vi "test_F9P_232-2.vi"() -> ()   [LabVIEW 2019] (continued)
1*73\r\n$GBGSV,5,4,17,16,25,186,30,27,11,317,,28,62,307,37,33,76,249,24,1*7B\r\n$GBGSV,5,5,17,34,10,143,,1*40\r\n$GBGSV,5,1,17,01,42,153,,03,45,207,,04,35,133,,05,09,257,,3*7E\r\n$GBGSV,5,2,17,06,29,183,,07,07,201,,08,66,358,42,09,09,195,,3*7C\r\n$GBGSV,5,3,17,10,14,222,,11,34,144,,13,51,316,,14,73,036,46,3*70\r\n$GBGSV,5,4,17,16,25,186,33,27,11,317,,28,62,307,,33,76,249,,3*78\r\n$GBGSV,5,5,17,34,10,143,,3*42\r\n$GNGLL,3723.59652,N,12656.92463,E,065255.00,A,A*72\r\n$GNRMC,065256.00,A,3723.59660,N,12656.92463,E,0.025,,250720,,,A,V*16\r\n$GNVTG,,T,,M,0.025,N,0.047,K,A*39\r\n$GNGGA,065256.00,3723.59660,N,12656.92463,E,1,12,0.80,36.1,M,18.5,M,,*76\r\n$GNGSA,A,3,29,17,19,06,12,05,02,09,,,,,1.28,0.80,1.01,1*0C\r\n$GNGSA,A,3,85,71,72,,,,,,,,,,1.28,0.80,1.01,2*0F\r\n$GNGSA,A,3,36,19,11,04,09,12,,,,,,,1.28,0.80,1.01,3*03\r\n$GNGSA,A,3,28,11,14,10,33,08,,,,,,,1.28,0.80,1.01,4*01\r\n$GPGSV,4,1,13,02,69,341,33,04,05,036,09,05,51,267,38,06,55,084,32,1*67\r\n$GPGSV,4,2,13,07,08,101,,09,35,053,36,12,16,259,29,13,12,191,,1*6A\r\n$GPGSV,4,3,13,17,14,158,15,19,32,163,36,25,10,289,21,29,11,322,19,1*64\r\n$GPGSV,4,4,13,30,04,130,,1*53\r\n$GPGSV,4,1,13,02,69,341,,04,05,036,,05,51,267,34,06,55,084,34,6*63\r\n$GPGSV,4,2,13,07,08,101,19,09,35,053,36,12,16,259,,13,12,191,,6*6E\r\n$GPGSV,4,3,13,17,14,158,,19,32,163,,25,10,289,13,29,11,322,,6*6B\r\n$GPGSV,4,4,13,30,04,130,,6*54\r\n$GLGSV,2,1,06,70,49,030,,71,73,235,35,72,22,219,31,84,04,137,11,1*74\r\n$GLGSV,2,2,06,85,59,121,30,86,57,339,,1*7B\r\n$GLGSV,2,1,06,70,49,030,,71,73,235,40,72,22,219,16,84,04,137,12,3*72\r\n$GLGSV,2,2,06,85,59,121,33,86,57,339,,3*7A\r\n$GAGSV,3,1,09,02,02,284,09,04,67,075,28,05,01,213,,09,48,198,36,7*76\r\n$GAGSV,3,2,09,11,78,057,26,12,29,118,16,18,59,273,42,19,15,041,19,7*71\r\n$GAGSV,3,3,09,36,38,315,26,7*47\r\n$GAGSV,3,1,09,02,02,284,,04,67,075,40,05,01,213,,09,48,198,34,2*76\r\n$GAGSV,3,2,09,11,78,057,35,12,29,118,25,18,59,273,33,19,15,041,,2*78\r\n$GAGSV,3,3,09,36,38,315,17,2*40\r\n$GBGSV,5,1,17,01,42,153,,03,45,207,,04,35,133,,05,09,257,,1*7C\r\n$GBGSV,5,2,17,06,29,183,,07,07,201,,08,66,358,34,09,09,195,,1*7F\r\n$GBGSV,5,3,17,10,14,222,23,11,34,144,25,13,51,316,,14,73,036,35,1*70\r\n$GBGSV,5,4,17,16,25,186,30,27,11,317,,28,62,307,37,33,76,249,27,1*78\r\n$GBGSV,5,5,17,34,10,143,,1*40\r\n$GBGSV,5,1,17,01,42,153,,03,45,207,,04,35,133,,05,09,257,,3*7E\r\n$GBGSV,5,2,17,06,29,183,,07,07,201,,08,66,358,41,09,09,195,,3*7F\r\n$GBGSV,5,3,17,10,14,222,,11,34,144,,13,51,316,,14,73,036,44,3*72\r\n$GBGSV,5,4,17,16,25,186,32,27,11,317,,28,62,307,,33,76,249,,3*79\r\n$GBGSV,5,5,17,34,10,143,,3*42\r\n$GNGLL,3723.59660,N,12656.92463,E,065256.00,A,A*70\r\n$GNRMC,065257.00,A,3723.59674,N,12656.92461,E,0.007,,250720,,,A,V*10\r\n$GNVTG,,T,,M,0.007,N,0.013,K,A*38\r\n$GNGGA,065257.00,3723.59674,N,12656.92461,E,1,12,0.70,36.5,M,18.5,M,,*7B\r\n$GNGSA,A,3,29,17,19,06,12,05,02,09,,,,,1.18,0.70,0.95,1*0C\r\n$GNGSA,A,3,85,71,72,,,,,,,,,,1.18,0.70,0.95,2*0F\r\n$GNGSA,A,3,36,19,11,04,09,12,,,,,,,1.18,0.70,0.95,3*03\r\n$GNGSA,A,3,28,11,14,10,33,08,,,,,,,1.18,0.70,0.95,4*01\r\n$GPGSV,4,1,13,02,69,341,37,04,05,036,10,05,51,267,37,06,55,084,32,1*64\r\n$GPGSV,4,2,13,07,08,101,,09,35,053,36,12,16,259,29,13,12,191,,1*6A\r\n$GPGSV,4,3,13,17,14,158,15,19,32,163,36,25,10,289,21,29,11,322,19,1*64\r\n$GPGSV,4,4,13,30,04,130,,1*53\r\n$GPGSV,4,1,13,02,69,341,,04,05,036,,05,51,267,33,06,55,084,32,6*62\r\n$GPGSV,4,2,13,07,08,101,15,09,35,053,35,12,16,259,,13,12,191,,6*61\r\n$GPGSV,4,3,13,17,14,158,,19,32,163,,25,10,289,15,29,11,322,,6*6D\r\n$GPGSV,4,4,13,30,04,130,,6*54\r\n$GLGSV,2,1,06,70,49,030,,71,73,235,35,72,22,219,31,84,04,137,06,1*72\r\n$GLGSV,2,2,06,85,59,121,29,86,57,339,,1*73\r\n$GLGSV,2,1,06,70,49,030,,71,73,235,40,72,22,219,10,84,04,137,10,3*76\r\n$GLGSV,2,2,06,85,59,121,32,86,57,339,,3*7B\r\n$GAGSV,3,1,09,02,02,284,08,04,67,075,29,05,01,213,,09,48,198,36,7*76\r\n$GAGSV,3,2,09,11,78,057,26,12,29,118,16,18,59,273,42,19,14,041,19,7*70\r\n$GAGSV,3,3,09,36,38,315,26,7*47\r\n$GAGSV,3,1,09,02,02,284,,04,67,075,39,05,01,213,,09,48,198,34,2*78\r\n$GAGSV,3,2,09,11,78,057,34,12,29,118,26,18,59,273,34,19,14,041,,2*7C\r\n$GAGSV,3,3,09,36,38,315,18,2*4F\r\n$GBGSV,5,1,17,01,42,153,,03,45,207,,04,35,133,,05,09,257,,1*7C\r\n$GBGSV,5,2,17,06,29,183,,07,07,201,,08,66,358,34,09,09,195,,1*7F\r\n$GBGSV,5,3,17,10,14,222,23,11,34,144,25,13,51,316,,14,73,036,35,1*70\r\n$GBGSV,5,4,17,16,25,186,30,27,11,317,,28,62,307,37,33,76,249,29,1*76\r\n$GBGSV,5,5,17,34,10,143,,1*40\r\n$GBGSV,5,1,17,01,42,153,,03,45,207,,04,35,133,,05,09,257,,3*7E\r\n$GBGSV,5,2,17,06,29,183,,07,07,201,,08,66,358,40,09,09,195,,3*7E\r\n$GBGSV,5,3,17,10,14,222,,11,34,144,28,13,51,316,,14,73,036,42,3*7E\r\n$GBGSV,5,4,17,16,25,186,32,27,11,317,,28,62,307,,33,76,249,,3*79\r\n$GBGSV,5,5,17,34,10,143,,3*42\r\n$GNGLL,3723.59674,N,12656.92461,E,065257.00,A,A*76\r\n$GNRMC,065258.00,A,3723.59689,N,12656.92458,E,0.035,,250720,,,A,V*16\r\n$GNVTG,,T,,M,0.035,N,0.065,K,A*38\r\n$GNGGA,065258.00,3723.59689,N,12656.92458,E,1,12,0.70,37.0,M,18.5,M,,*78\r\n$GNGSA,A,3,29,17,19,06,12,05,02,09,,,,,1.18,0.70,0.95,1*0C\r\n$GNGSA,A,3,85,71,72,,,,,,,,,,1.18,0.70,0.95,2*0F\r\n$GNGSA,A,3,36,19,11,04,09,12,,,,,,,1.18,0.70,0.95,3*03\r\n$GNGSA,A,3,28,11,14,10,33,08,,,,,,,1.18,0.70,0.95,4*01\r\n$GPGSV,4,1,13,02,69,341,37,04,05,036,10,05,51,267,37,06,55,084,32,1*64\r\n$GPGSV,4,2,13,07,08,101,,09,35,053,35,12,16,259,29,13,12,191,,1*69\r\n$GPGSV,4,3,13,17,14,158,15,19,32,163,36,25,10,289,21,29,11,322,20,1*6E\r\n$GPGSV,4,4,13,30,04,130,,1*53\r\n$GPGSV,4,1,13,02,69,341,,04,05,036,,05,51,267,33,06,55,084,32,6*62\r\n$GPGSV,4,2,13,07,08,101,,09,35,053,35,12,16,259,,13,12,191,,6*65\r\n$GPGSV,4,3,13,17,14,158,,19,32,163,,25,10,289,15,29,11,322,,6*6D\r\n$GPGSV,4,4,13,30,04,130,,6*54\r\n$GLGSV,2,1,06,70,49,030,,71,73,235,35,72,22,219,31,84,04,137,06,1*72\r\n$GLGSV,2,2,06,85,59,121,26,86,57,339,,1*7C\r\n$GLGSV,2,1,06,70,49,030,,71,73,235,38,72,22,219,10,84,04,137,10,3*79\r\n$GLGSV,2,2,06,85,59,121,31,86,57,339,,3*78\r\n$GAGSV,3,1,09,02,02,284,09,04,67,075,29,05,01,213,,09,48,198,36,7*77\r\n$GAGSV,3,2,09,11,78,057,26,12,29,118,16,18,59,273,42,19,14,041,18,7*71\r\n$GAGSV,3,3,09,36,38,315,25,7*44\r\n$GAGSV,3,1,09,02,02,284,,04,67,075,39,05,01,213,,09,48,198,34,2*78\r\n$GAGSV,3,2,09,11,78,057,37,12,29,118,27,18,59,273,34,19,14,041,,2*7E\r\n$GAGSV,3,3,09,36,38,315,17,2*40\r\n$GBGSV,5,1,17,01,42,153,,03,45,207,,04,35,133,,05,09,257,,1*7C\r\n$GBGSV,5,2,17,06,29,183,,07,07,201,,08,66,358,34,09,09,195,,1*7F\r\n$GBGSV,5,3,17,10,14,222,23,11,34,144,25,13,51,316,,14,73,036,35,1*70\r\n$GBGSV,5,4,17,16,25,186,31,27,11,317,,28,62,307,37,33,76,249,29,1*77\r\n$GBGSV,5,5,17,34,10,143,,1*40\r\n$GBGSV,5,1,17,01,42,153,,03,45,207,,04,35,133,,05,09,257,,3*7E\r\n$GBGSV,5,2,17,06,29,183,,07,07,201,,08,66,358,40,09,09,195,,3*7E\r\n$GBGSV,5,3,17,10,14,222,,11,34,144,28,13,51,316,,14,73,036,42,3*7E\r\n$GBGSV,5,4,17,16,25,186,32,27,11,317,,28,62,307,,33,76,249,,3*79\r\n$GBGSV,5,5,17,34,10,143,,3*42\r\n$GNGLL,3723.59689,N,12656.92458,E,065258.00,A,A*71\r\n$GNRMC,065259.00,A,3723.59709,N,12656.92456,E,0.071,,250720,,,A,V*10\r\n$GNVTG,,T,,M,0.071,N,0.132,K,A*3B\r\n$GNGGA,065259.00,3723.59709,N,12656.92456,E,1,12,0.70,37.6,M,18.5,M,,*78\r\n$GNGSA,A,3,29,17,19,06,12,05,02,09,,,,,1.18,0.70,0.95,1*0C\r\n$GNGSA,A,3,85,71,72,,,,,,,,,,1.18,0.70,0.95,2*0F\r\n$GNGSA,A,3,36,19,11,04,09,12,,,,,,,1.18,0.70,0.95,3*03\r\n$GNGSA,A,3,28,11,14,10,33,08,,,,,,,1.18,0.70,0.95,4*01\r\n$GPGSV,4,1,13,02,69,341,36,04,05,036,12,05,51,267,37,06,55,084,32,1*67\r\n$GPGSV,4,2,13,07,08,101,,09,35,053,35,12,16,259,29,13,12,191,,1*69\r\n$GPGSV,4,3,13,17,14,158,15,19,32,163,36,25,10,289,20,29,11,322,19,1*65\r\n$GPGSV,4,4,13,30,04,130,,1*53\r\n$GPGSV,4,1,13,02,69,341,,04,05,036,,05,51,267,33,06,55,084,33,6*63\r\n$GPGSV,4,2,13,07,08,101,,09,35,053,35,12,16,259,,13,12,191,,6*65\r\n$GPGSV,4,3,13,17,14,158,,19,32,163,,25,10,289,15,29,11,322,,6*6D\r\n$GPGSV,4,4,13,30,04,130,,6*54\r\n$GLGSV,2,1,06,70,49,030,,71,73,235,35,72,22,219,31,84,04,137,12,1*77\r\n$GLGSV,2,2,06,85,59,121,23,86,57,339,,1*79\r\n$GLGSV,2,1,06,70,49,030,,71,73,235,38,72,22,219,14,84,04,137,10,3*7D\r\n$GLGSV,2,2,06,85,59,121,30,86,57,339,,3*79\r\n$GAGSV,3,1,09,02,02,284,09,04,67,075,29,05,01,213,,09,48,198,36,7*77\r\n$GAGSV,3,2,09,11,78,057,26,12,29,118,16,18,59,273,42,19,14,041,19,7*70\r\n$GAGSV,3,3,09,36,38,315,25,7*44\r\n$GAGSV,3,1,09,02,02,284,,04,67,075,39,05,01,213,,09,48,198,34,2*78\r\n$GAGSV,3,2,09,11,78,057,37,12,29,118,27,18,59,273,34,19,14,041,,2*7E\r\n$GAGSV,3,3,09,36,38,315,17,2*40\r\n$GBGSV,5,1,17,01,42,153,,03,45,207,,04,35,133,,05,09,257,,1*7C\r\n$GBGSV,5,2,17,06,29,183,,07,07,201,,08,66,358,34,09,09,195,,1*7F\r\n$GBGSV,5,3,17,10,14,222,24,11,34,144,25,13,51,316,,14,73,036,35,1*77\r\n$GBGSV,5,4,17,16,25,186,31,27,11,317,,28,62,307,37,33,76,249,28,1*76\r\n$GBGSV,5,5,17,34,10,143,,1*40\r\n$GBGSV,5,1,17,01,42,153,,03,45,207,,04,35,133,,05,09,257,,3*7E\r\n$GBGSV,5,2,17,06,29,183,,07,07,201,,08,66,358,40,09,09,195,,3*7E\r\n$GBGSV,5,3,17,10,14,222,,11,34,144,28,13,51,316,,14,73,036,43,3*7F\r\n$GBGSV,5,4,17,16,25,186,32,27,11,317,,28,62,307,,33,76,249,,3*79\r\n$GBGSV,5,5,17,34,10,143,,3*42\r\n$GNGLL,3723.59709,N,12656.92456,E,065259.00,A,A*77\r\n$GNRMC,065300.00,A,3723.59721,N,12656.92455,E,0.021,,250720,,,A,V*11\r\n$GNVTG,,T,,M,0.021,N,0.039,K,A*34\r\n$GNGGA,065300.00,3723.59721,N,12656.92455,E,1,12,0.78,38.0,M,18.5,M,,*7D\r\n$GNGSA,A,3,29,17,19,06,12,05,02,09,,,,,1.20,0.78,0.92,1*08\r\n$GNGSA,A,3,85,71,72,,,,,,,,,,1.20,0.78,0.92,2*0B\r\n$GNGSA,A,3,36,19,11,04,09,12,,,,,,,1.20,0.78,0.92,3*07\r\n$GNGSA,A,3,28,11,14,10,33,08,,,,,,,1.20,0.78,0.92,4*05\r\n$GPGSV,4,1,13,02,69,341,36,04,05,036,07,05,51,267,37,06,55,084,32,1*63\r\n$GPGSV,4,2,13,07,08,101,,09,35,053,35,12,16,259,28,13,12,191,,1*68\r\n$GPGSV,4,3,13,17,14,158,16,19,32,163,36,25,10,289,20,29,11,322,20,1*6C\r\n$GPGSV,4,4,13,30,04,130,,1*53\r\n$GPGSV,4,1,13,02,69,341,,04,05,036,,05,51,267,32,06,55,084,32,6*63\r\n$GPGSV,4,2,13,07,08,101,,09,35,053,32,12,16,259,,13,12,191,,6*62\r\n$GPGSV,4,3,13,17,14,158,,19,32,163,,25,10,289,15,29,11,322,,6*6D\r\n$GPGSV,4,4,13,30,04,130,,6*54\r\n$GLGSV,2,1,06,70,49,030,,71,73,235,35,72,22,219,31,84,04,137,09,1*7D\r\n$GLGSV,2,2,06,85,59,121,18,86,57,339,,1*71\r\n$GLGSV,2,1,06,70,49,030,,71,73,235,38,72,22,219,15,84,04,137,09,3*74\r\n$GLGSV,2,2,06,85,59,121,30,86,57,339,,3*79\r\n$GAGSV,3,1,09,02,02,284,09,04,67,075,30,05,01,213,,09,48,198,36,7*7F\r\n$GAGSV,3,2,09,11,78,057,26,12,29,118,18,18,59,273,43,19,14,041,18,7*7E\r\n$GAGSV,3,3,09,36,38,315,26,7*47\r\n$GAGSV,3,1,09,02,02,284,,04,67,075,39,05,01,213,,09,48,198,33,2*7F\r\n$GAGSV,3,2,09,11,78,057,35,12,29,118,28,18,59,273,35,19,14,041,,2*72\r\n$GAGSV,3,3,09,36,38,315,16,2*41\r\n$GBGSV,5,1,17,01,42,153,,03,45,207,,04,35,133,,05,09,257,,1*7C\r\n$GBGSV,5,2,17,06,29,183,,07,07,201,,08,66,358,34,09,09,195,,1*7F\r\n$GBGSV,5,3,17,10,14,222,23,11,34,144,25,13,51,316,,14,73,036,35,1*70\r\n$GBGSV,5,4,17,16,25,186,31,27,11,317,,28,62,307,37,33,76,249,28,1*76\r\n$GBGSV,5,5,17,34,10,143,,1*40\r\n$GBGSV,5,1,17,01,42,153,,03,45,207,,04,35,133,,05,09,257,,3*7E\r\n$GBGSV,5,2,17,06,29,183,,07,07,201,,08,66,358,39,09,09,195,,3*70\r\n$GBGSV,5,3,17,10,14,222,,11,34,144,28,13,51,316,,14,73,036,40,3*7C\r\n$GBGSV,5,4,17,16,25,186,31,27,11,317,,28,62,307,,33,76,249,,3*7A\r\n$GBGSV,5,5,17,34,10,143,,3*42\r\n$GNGLL,3723.59721,N,12656.92455,E,065300.00,A,A*73\r\n$GNRMC,065301.00,A,3723.59736,N,12656.92455,E,0.032,,250720,,,A,V*14\r\n$GNVTG,,T,,M,0.032,N,0.059,K,A*30\r\n$GNGGA,065301.00,3723.59736,N,12656.92455,E,1,12,0.72,38.4,M,18.5,M,,*74\r\n$GNGSA,A,3,29,17,19,06,12,05,02,09,,,,,1.15,0.72,0.90,1*06\r\n$GNGSA,A,3,85,71,72,,,,,,,,,,1.15,0.72,0.90,2*05\r\n$GNGSA,A,3,36,19,11,04,09,12,,,,,,,1.15,0.72,0.90,3*09\r\n$GNGSA,A,3,28,11,14,10,33,08,,,,,,,1.15,0.72,0.90,4*0B\r\n$GPGSV,4,1,13,02,69,341,33,04,05,036,08,05,51,267,37,06,55,084,33,1*68\r\n$GPGSV,4,2,13,07,08,101,,09,35,053,35,12,16,259,28,13,12,191,,1*68\r\n$GPGSV,4,3,13,17,14,158,15,19,32,163,36,25,10,289,21,29,11,322,21,1*6F\r\n$GPGSV,4,4,13,30,04,130,,1*53\r\n$GPGSV,4,1,13,02,69,341,,04,05,036,,05,51,267,33,06,55,084,35,6*65\r\n$GPGSV,4,2,13,07,08,101,,09,35,053,37,12,16,259,,13,12,191,,6*67\r\n$GPGSV,4,3,13,17,14,158,,19,32,163,,25,10,289,16,29,11,322,,6*6E\r\n$GPGSV,4,4,13,30,04,130,,6*54\r\n$GLGSV,2,1,06,70,49,030,,71,73,235,35,72,22,219,31,84,04,137,08,1*7C\r\n$GLGSV,2,2,06,85,59,121,17,86,57,339,,1*7E\r\n$GLGSV,2,1,06,70,49,030,,71,73,235,38,72,22,219,18,84,04,137,11,3*70\r\n$GLGSV,2,2,06,85,59,121,30,86,57,339,,3*79\r\n$GAGSV,3,1,09,02,02,284,11,04,67,075,30,05,01,213,,09,48,198,36,7*76\r\n$GAGSV,3,2,09,11,78,057,26,12,29,118,18,18,59,273,43,19,14,041,19,7*7F\r\n$GAGSV,3,3,09,36,38,315,26,7*47\r\n$GAGSV,3,1,09,02,02,284,,04,67,075,39,05,01,213,,09,48,198,33,2*7F\r\n$GAGSV,3,2,09,11,78,057,35,12,29,118,27,18,59,273,34,19,14,041,,2*7C\r\n$GAGSV,3,3,09,36,38,315,15,2*42\r\n$GBGSV,5,1,17,01,42,153,,03,45,207,,04,35,133,,05,09,257,,1*7C\r\n$GBGSV,5,2,17,06,29,183,,07,07,201,,08,66,358,33,09,09,195,,1*78\r\n$GBGSV,5,3,17,10,14,222,24,11,34,144,25,13,51,316,,14,73,036,35,1*77\r\n$GBGSV,5,4,17,16,25,186,31,27,11,317,,28,62,307,36,33,76,249,29,1*76\r\n$GBGSV,5,5,17,34,10,143,,1*40\r\n$GBGSV,5,1,17,01,42,153,,03,45,207,,04,35,133,,05,09,257,,3*7E\r\n$GBGSV,5,2,17,06,29,183,,07,07,201,,08,66,358,39,09,09,195,,3*70\r\n$GBGSV,5,3,17,10,14,222,,11,34,144,27,13,51,316,,14,73,036,43,3*70\r\n$GBGSV,5,4,17,16,25,186,31,27,11,317,,28,62,307,,33,76,249,,3*7A\r\n$GBGSV,5,5,17,34,10,143,,3*42\r\n$GNGLL,3723.59736,N,12656.92455,E,065301.00,A,A*74\r\n$GNRMC,065302.00,A,3723.59754,N,12656.92453,E,0.052,,250720,,,A,V*13\r\n$GNVTG,,T,,M,0.052,N,0.096,K,A*35\r\n$GNGGA,065302.00,3723.59754,N,12656.92453,E,1,12,0.72,38.8,M,18.5,M,,*79\r\n$GNGSA,A,3,29,17,19,06,12,05,02,09,,,,,1.15,0.72,0.90,1*06\r\n$GNGSA,A,3,85,71,72,,,,,,,,,,1.15,0.72,0.90,2*05\r\n$GNGSA,A,3,36,19,11,04,09,12,,,,,,,1.15,0.72,0.90,3*09\r\n$GNGSA,A,3,28,11,14,10,33,08,,,,,,,1.15,0.72,0.90,4*0B\r\n$GPGSV,4,1,13,02,69,341,34,04,05,036,08,05,51,267,37,06,55,084,33,1*6F\r\n$GPGSV,4,2,13,07,08,101,,09,35,053,35,12,16,259,28,13,12,191,,1*68\r\n$GPGSV,4,3,13,17,14,158,14,19,32,163,36,25,10,289,22,29,11,322,21,1*6D\r\n$GPGSV,4,4,13,30,04,130,,1*53\r\n$GPGSV,4,1,13,02,69,341,,04,05,036,,05,51,267,32,06,55,084,31,6*60\r\n$GPGSV,4,2,13,07,08,101,,09,35,053,34,12,16,259,,13,12,191,,6*64\r\n$GPGSV,4,3,13,17,14,158,,19,32,163,,25,10,289,16,29,11,322,,6*6E\r\n$GPGSV,4,4,13,30,04,130,,6*54\r\n$GLGSV,2,1,06,70,49,030,,71,73,235,35,72,22,219,31,84,04,137,08,1*7C\r\n$GLGSV,2,2,06,85,59,121,21,86,57,339,,1*7B\r\n$GLGSV,2,1,06,70,49,030,,71,73,235,36,72,22,219,19,84,04,137,10,3*7E\r\n$GLGSV,2,2,06,85,59,121,29,86,57,339,,3*71\r\n$GAGSV,3,1,09,02,02,284,08,04,67,075,29,05,01,213,,09,48,198,36,7*76\r\n$GAGSV,3,2,09,11,78,057,26,12,29,118,19,18,59,273,43,19,14,041,19,7*7E\r\n$GAGSV,3,3,09,36,38,315,26,7*47\r\n$GAGSV,3,1,09,02,02,284,,04,67,075,38,05,01,213,,09,48,198,34,2*79\r\n$GAGSV,3,2,09,11,78,057,36,12,29,118,28,18,59,273,31,19,14,041,,2*75\r\n$GAGSV,3,3,09,36,38,315,16,2*41\r\n$GBGSV,5,1,17,01,42,153,,03,45,207,,04,35,133,,05,09,257,,1*7C\r\n$GBGSV,5,2,17,06,29,183,,07,07,201,,08,66,358,33,09,09,195,,1*78\r\n$GBGSV,5,3,17,10,14,222,24,11,34,144,24,13,51,316,,14,73,036,35,1*76\r\n$GBGSV,5,4,17,16,25,186,31,27,11,317,,28,62,307,37,33,76,249,28,1*76\r\n$GBGSV,5,5,17,34,10,143,,1*40\r\n$GBGSV,5,1,17,01,42,153,,03,45,207,,04,35,133,,05,09,257,,3*7E\r\n$GBGSV,5,2,17,06,29,183,,07,07,201,,08,66,358,38,09,09,195,,3*71\r\n$GBGSV,5,3,17,10,14,222,,11,34,144,27,13,51,316,,14,73,036,41,3*72\r\n$GBGSV,5,4,17,16,25,186,31,27,11,317,,28,62,307,,33,76,249,,3*7A\r\n$GBGSV,5,5,17,34,10,143,,3*42\r\n$GNGLL,3723.59754,N,12656.92453,E,065302.00,A,A*75\r\n$GNRMC,065303.00,A,3723.59771,N,12656.92452,E,0.013,,250720,,,A,V*11\r\n$GNVTG,,T,,M,0.013,N,0.023,K,A*3E\r\n$GNGGA,065303.00,3723.59771,N,12656.92452,E,1,12,0.72,39.1,M,18.5,M,,*76\r\n$GNGSA,A,3,29,17,19,06,12,05,02,09,,,,,1.15,0.72,0.90,1*06\r\n$GNGSA,A,3,85,71,72,,,,,,,,,,1.15,0.72,0.90,2*05\r\n$GNGSA,A,3,36,19,11,04,09,12,,,,,,,1.15,0.72,0.90,3*09\r\n$GNGSA,A,3,28,11,14,10,33,08,,,,,,,1.15,0.72,0.90,4*0B\r\n$GPGSV,4,1,13,02,69,341,33,04,05,036,09,05,51,267,38,06,55,084,33,1*66\r\n$GPGSV,4,2,13,07,08,101,,09,35,053,35,12,16,259,27,13,12,191,,1*67\r\n$GPGSV,4,3,13,17,14,158,14,19,32,163,36,25,10,289,22,29,11,322,22,1*6E\r\n$GPGSV,4,4,13,30,04,130,,1*53\r\n$GPGSV,4,1,13,02,69,341,,04,05,036,,05,51,267,32,06,55,084,37,6*66\r\n$GPGSV,4,2,13,07,08,101,,09,35,053,37,12,16,259,,13,12,191,,6*67\r\n$GPGSV,4,3,13,17,14,158,,19,32,163,,25,10,289,16,29,11,322,,6*6E\r\n$GPGSV,4,4,13,30,04,130,,6*54\r\n$GLGSV,2,1,06,70,49,030,,71,73,235,36,72,22,219,31,84,04,137,11,1*77\r\n$GLGSV,2,2,06,85,59,121,25,86,57,339,,1*7F\r\n$GLGSV,2,1,06,70,49,030,,71,73,235,37,72,22,219,13,84,04,137,09,3*7D\r\n$GLGSV,2,2,06,85,59,121,28,86,57,339,,3*70\r\n$GAGSV,3,1,09,02,02,284,07,04,67,075,29,05,01,213,,09,48,198,36,7*79\r\n$GAGSV,3,2,09,11,78,057,26,12,29,118,21,18,59,273,43,19,14,041,18,7*74\r\n$GAGSV,3,3,09,36,38,315,26,7*47\r\n$GAGSV,3,1,09,02,02,284,,04,67,075,40,05,01,213,,09,48,198,33,2*71\r\n$GAGSV,3,2,09,11,78,057,36,12,29,118,28,18,59,273,32,19,14,041,,2*76\r\n$GAGSV,3,3,09,36,38,315,17,2*40\r\n$GBGSV,5,1,17,01,42,153,,03,45,207,,04,35,133,,05,09,257,,1*7C\r\n$GBGSV,5,2,17,06,29,183,,07,07,201,,08,66,358,33,09,09,195,,1*78\r\n$GBGSV,5,3,17,10,14,222,23,11,34,144,23,13,51,316,,14,73,036,35,1*76\r\n$GBGSV,5,4,17,16,25,186,31,27,11,317,,28,62,307,37,33,76,249,29,1*77\r\n$GBGSV,5,5,17,34,10,143,,1*40\r\n$GBGSV,5,1,17,01,42,153,,03,45,207,,04,35,133,,05,09,257,,3*7E\r\n$GBGSV,5,2,17,06,29,183,,07,07,201,,08,66,358,39,09,09,195,,3*70\r\n$GBGSV,5,3,17,10,14,222,,11,34,144,27,13,51,316,,14,73,036,43,3*70\r\n$GBGSV,5,4,17,16,25,186,32,27,11,317,,28,62,307,,33,76,249,,3*79\r\n$GBGSV,5,5,17,34,10,143,,3*42\r\n$GNGLL,3723.59771,N,12656.92452,E,065303.00,A,A*72\r\n$GNRMC,065304.00,A,3723.59784,N,12656.92450,E,0.021,,250720,,,A,V*1F\r\n$GNVTG,,T,,M,0.021,N,0.039,K,A*34\r\n$GNGGA,065304.00,3723.59784,N,12656.92450,E,1,12,0.78,39.4,M,18.5,M,,*76\r\n$GNGSA,A,3,29,17,19,06,12,05,02,09,,,,,1.20,0.78,0.92,1*08\r\n$GNGSA,A,3,85,71,72,,,,,,,,,,1.20,0.78,0.92,2*0B\r\n$GNGSA,A,3,36,19,11,04,09,12,,,,,,,1.20,0.78,0.92,3*07\r\n$GNGSA,A,3,28,11,14,10,33,08,,,,,,,1.20,0.78,0.92,4*05\r\n$GPGSV,4,1,13,02,69,341,33,04,05,036,09,05,51,267,38,06,55,084,33,1*66\r\n$GPGSV,4,2,13,07,08,101,,09,35,053,35,12,16,259,27,13,12,191,,1*67\r\n$GPGSV,4,3,13,17,14,158,13,19,32,163,36,25,10,289,22,29,11,322,22,1*69\r\n$GPGSV,4,4,13,30,04,130,,1*53\r\n$GPGSV,4,1,13,02,69,341,,04,05,036,,05,51,267,33,06,55,084,34,6*64\r\n$GPGSV,4,2,13,07,08,101,,09,35,053,37,12,16,259,,13,12,191,,6*67\r\n$GPGSV,4,3,13,17,14,158,,19,32,163,,25,10,289,17,29,11,322,,6*6F\r\n$GPGSV,4,4,13,30,04,130,,6*54\r\n$GLGSV,2,1,06,70,49,030,,71,73,235,35,72,22,219,30,84,04,137,09,1*7C\r\n$GLGSV,2,2,06,85,59,121,27,86,57,339,,1*7D\r\n$GLGSV,2,1,06,70,49,030,,71,73,235,37,72,22,219,16,84,04,137,08,3*79\r\n$GLGSV,2,2,06,85,59,121,28,86,57,339,,3*70\r\n$GAGSV,3,1,09,02,02,284,08,04,67,075,29,05,01,213,,09,48,198,36,7*76\r\n$GAGSV,3,2,09,11,78,057,26,12,29,118,22,18,59,273,43,19,14,041,18,7*77\r\n$GAGSV,3,3,09,36,38,315,26,7*47\r\n$GAGSV,3,1,09,02,02,284,,04,67,075,40,05,01,213,,09,48,198,33,2*71\r\n$GAGSV,3,2,09,11,78,057,36,12,29,118,27,18,59,273,32,19,14,041,,2*79\r\n$GAGSV,3,3,09,36,38,315,18,2*4F\r\n$GBGSV,5,1,17,01,42,153,,03,45,207,,04,35,133,,05,09,257,,1*7C\r\n$GBGSV,5,2,17,06,29,183,,07,07,201,,08,66,358,33,09,09,195,,1*78\r\n$GBGSV,5,3,17,10,14,222,23,11,34,144,23,13,51,316,,14,73,036,35,1*76\r\n$GBGSV,5,4,17,16,25,186,31,27,11,317,,28,62,307,37,33,76,249,29,1*77\r\n$GBGSV,5,5,17,34,10,143,,1*40\r\n$GBGSV,5,1,17,01,42,153,,03,45,207,,04,35,133,,05,09,257,,3*7E\r\n$GBGSV,5,2,17,06,29,183,,07,07,201,,08,66,358,40,09,09,195,,3*7E\r\n$GBGSV,5,3,17,10,14,222,,11,34,144,27,13,51,316,,14,73,036,43,3*70\r\n$GBGSV,5,4,17,16,25,186,32,27,11,317,,28,62,307,,33,76,249,,3*79\r\n$GBGSV,5,5,17,34,10,143,,3*42\r\n$GNGLL,3723.59784,N,12656.92450,E,065304.00,A,A*7D\r\n$GNRMC,065305.00,A,3723.59802,N,12656.92448,E,0.045,,250720,,,A,V*14\r\n$GNVTG,,T,,M,0.045,N,0.084,K,A*30\r\n$GNGGA,065305.00,3723.59802,N,12656.92448,E,1,12,0.72,39.8,M,18.5,M,,*79\r\n$GNGSA,A,3,29,17,19,06,12,05,02,09,,,,,1.15,0.72,0.90,1*06\r\n$GNGSA,A,3,85,71,72,,,,,,,,,,1.15,0.72,0.90,2*05\r\n$GNGSA,A,3,36,19,11,04,09,12,,,,,,,1.15,0.72,0.90,3*09\r\n$GNGSA,A,3,28,11,14,10,33,08,,,,,,,1.15,0.72,0.90,4*0B\r\n$GPGSV,4,1,13,02,69,341,36,04,05,036,11,05,51,267,38,06,55,084,34,1*6D\r\n$GPGSV,4,2,13,07,08,101,,09,35,053,35,12,16,259,26,13,12,191,17,1*60\r\n$GPGSV,4,3,13,17,14,158,14,19,32,163,36,25,10,289,22,29,11,322,22,1*6E\r\n$GPGSV,4,4,13,30,04,130,,1*53\r\n$GPGSV,4,1,13,02,69,341,,04,05,036,,05,51,267,33,06,55,084,32,6*62\r\n$GPGSV,4,2,13,07,08,101,,09,35,053,34,12,16,259,,13,12,191,,6*64\r\n$GPGSV,4,3,13,17,14,158,,19,32,163,,25,10,289,17,29,11,322,,6*6F\r\n$GPGSV,4,4,13,30,04,130,,6*54\r\n$GLGSV,2,1,06,70,49,030,,71,73,235,36,72,22,219,30,84,04,137,10,1*77\r\n$GLGSV,2,2,06,85,59,121,30,86,57,339,,1*7B\r\n$GLGSV,2,1,06,70,49,030,,71,73,235,37,72,22,219,18,84,04,137,08,3*77\r\n$GLGSV,2,2,06,85,59,121,29,86,57,339,,3*71\r\n$GAGSV,3,1,09,02,02,284,09,04,67,075,29,05,01,213,,09,48,198,36,7*77\r\n$GAGSV,3,2,09,11,78,057,27,12,29,118,23,18,59,273,43,19,14,041,17,7*78\r\n$GAGSV,3,3,09,36,38,315,27,7*46\r\n$GAGSV,3,1,09,02,02,284,,04,67,075,39,05,01,213,,09,48,198,33,2*7F\r\n$GAGSV,3,2,09,11,78,057,36,12,29,118,27,18,59,273,33,19,14,041,,2*78\r\n$GAGSV,3,3,09,36,38,315,18,2*4F\r\n$GBGSV,5,1,17,01,42,153,,03,45,207,,04,35,133,,05,09,257,,1*7C\r\n$GBGSV,5,2,17,06,29,183,,07,07,201,,08,66,358,33,09,09,195,,1*78\r\n$GBGSV,5,3,17,10,14,222,23,11,34,144,22,13,51,316,,14,73,036,35,1*77\r\n$GBGSV,5,4,17,16,25,186,31,27,11,317,,28,62,307,37,33,76,249,29,1*77\r\n$GBGSV,5,5,17,34,10,143,,1*40\r\n$GBGSV,5,1,17,01,42,153,,03,45,207,,04,35,133,,05,09,257,,3*7E\r\n$GBGSV,5,2,17,06,29,183,,07,07,201,,08,66,358,40,09,09,195,,3*7E\r\n$GBGSV,5,3,17,10,14,222,,11,34,144,28,13,51,316,,14,73,036,43,3*7F\r\n$GBGSV,5,4,17,16,25,186,32,27,11,317,,28,62,307,,33,76,249,,3*79\r\n$GBGSV,5,5,17,34,10,143,,3*42\r\n$GNGLL,3723.59802,N,12656.92448,E,065305.00,A,A*74\r\n$GNRMC,065306.00,A,3723.59821,N,12656.92443,E,0.051,,250720,,,A,V*18\r\n$GNVTG,,T,,M,0.051,N,0.094,K,A*34\r\n$GNGGA,065306.00,3723.59821,N,12656.92443,E,1,12,0.72,40.2,M,18.5,M,,*74\r\n$GNGSA,A,3,29,17,19,06,12,05,02,09,,,,,1.15,0.72,0.90,1*06\r\n$GNGSA,A,3,85,71,72,,,,,,,,,,1.15,0.72,0.90,2*05\r\n$GNGSA,A,3,36,19,11,04,09,12,,,,,,,1.15,0.72,0.90,3*09\r\n$GNGSA,A,3,28,11,14,10,33,08,,,,,,,1.15,0.72,0.90,4*0B\r\n$GPGSV,4,1,13,02,69,341,36,04,05,036,12,05,51,267,38,06,55,084,34,1*6E\r\n$GPGSV,4,2,13,07,08,101,,09,35,053,35,12,16,259,26,13,12,191,17,1*60\r\n$GPGSV,4,3,13,17,14,158,16,19,32,163,36,25,10,289,22,29,11,322,22,1*6C\r\n$GPGSV,4,4,13,30,04,130,,1*53\r\n$GPGSV,4,1,13,02,69,341,,04,05,036,,05,51,267,33,06,55,084,32,6*62\r\n$GPGSV,4,2,13,07,08,101,,09,35,053,35,12,16,259,,13,12,191,,6*65\r\n$GPGSV,4,3,13,17,14,158,,19,32,163,,25,10,289,17,29,11,322,,6*6F\r\n$GPGSV,4,4,13,30,04,130,,6*54\r\n$GLGSV,2,1,06,70,49,030,,71,73,235,36,72,22,219,30,84,04,137,11,1*76\r\n$GLGSV,2,2,06,85,59,121,31,86,57,339,,1*7A\r\n$GLGSV,2,1,06,70,49,030,,71,73,235,37,72,22,219,19,84,04,137,09,3*77\r\n$GLGSV,2,2,06,85,59,121,29,86,57,339,,3*71\r\n$GAGSV,3,1,09,02,02,284,07,04,67,075,29,05,01,213,,09,48,198,35,7*7A\r\n$GAGSV,3,2,09,11,78,057,27,12,29,118,25,18,59,273,43,19,14,041,18,7*71\r\n$GAGSV,3,3,09,36,38,315,26,7*47\r\n$GAGSV,3,1,09,02,02,284,,04,67,075,40,05,01,213,,09,48,198,33,2*71\r\n$GAGSV,3,2,09,11,78,057,36,12,29,118,27,18,59,273,33,19,14,041,,2*78\r\n$GAGSV,3,3,09,36,38,315,19,2*4E\r\n$GBGSV,5,1,17,01,42,153,,03,45,207,,04,35,133,,05,09,257,,1*7C\r\n$GBGSV,5,2,17,06,29,183,,07,07,201,,08,66,358,33,09,09,195,,1*78\r\n$GBGSV,5,3,17,10,14,222,23,11,34,144,22,13,51,316,,14,73,036,35,1*77\r\n$GBGSV,5,4,17,16,25,186,31,27,11,317,,28,62,307,38,33,76,249,28,1*79\r\n$GBGSV,5,5,17,34,10,143,,1*40\r\n$GBGSV,5,1,17,01,42,153,,03,45,207,,04,35,133,,05,09,257,,3*7E\r\n$GBGSV,5,2,17,06,29,183,,07,07,201,,08,66,358,40,09,09,195,,3*7E\r\n$GBGSV,5,3,17,10,14,222,,11,34,144,28,13,51,316,,14,73,036,43,3*7F\r\n$GBGSV,5,4,17,16,25,186,32,27,11,317,,28,62,307,,33,76,249,,3*79\r\n$GBGSV,5,5,17,34,10,143,,3*42\r\n$GNGLL,3723.59821,N,12656.92443,E,065306.00,A,A*7D\r\n$GNRMC,065307.00,A,3723.59840,N,12656.92439,E,0.036,,250720,,,A,V*12\r\n$GNVTG,,T,,M,0.036,N,0.066,K,A*38\r\n$GNGGA,065307.00,3723.59840,N,12656.92439,E,1,12,0.72,40.5,M,18.5,M,,*78\r\n$GNGSA,A,3,29,17,19,06,12,05,02,09,,,,,1.15,0.72,0.90,1*06\r\n$GNGSA,A,3,85,71,72,,,,,,,,,,1.15,0.72,0.90,2*05\r\n$GNGSA,A,3,36,19,11,04,09,12,,,,,,,1.15,0.72,0.90,3*09\r\n$GNGSA,A,3,28,11,14,10,33,08,,,,,,,1.15,0.72,0.90,4*0B\r\n$GPGSV,4,1,13,02,69,341,37,04,05,036,13,05,51,267,38,06,55,084,35,1*6F\r\n$GPGSV,4,2,13,07,08,101,,09,35,053,35,12,16,259,26,13,12,191,18,1*6F\r\n$GPGSV,4,3,13,17,14,158,16,19,32,163,36,25,10,289,22,29,11,322,23,1*6D\r\n$GPGSV,4,4,13,30,04,130,,1*53\r\n$GPGSV,4,1,13,02,69,341,,04,05,036,,05,51,267,33,06,55,084,34,6*64\r\n$GPGSV,4,2,13,07,08,101,,09,35,053,36,12,16,259,,13,12,191,,6*66\r\n$GPGSV,4,3,13,17,14,158,,19,32,163,,25,10,289,17,29,11,322,,6*6F\r\n$GPGSV,4,4,13,30,04,130,,6*54\r\n$GLGSV,2,1,06,70,49,030,,71,73,235,35,72,22,219,29,84,04,137,09,1*74\r\n$GLGSV,2,2,06,85,59,121,31,86,57,339,,1*7A\r\n$GLGSV,2,1,06,70,49,030,,71,73,235,40,72,22,219,20,84,04,137,10,3*75\r\n$GLGSV,2,2,06,85,59,121,30,86,57,339,,3*79\r\n$GAGSV,3,1,09,02,02,284,10,04,67,075,29,05,01,213,,09,48,198,35,7*7C\r\n$GAGSV,3,2,09,11,78,057,27,12,29,118,25,18,59,273,43,19,14,041,17,7*7E\r\n$GAGSV,3,3,09,36,38,315,27,7*46\r\n$GAGSV,3,1,09,02,02,284,,04,67,075,39,05,01,213,,09,48,198,33,2*7F\r\n$GAGSV,3,2,09,11,78,057,35,12,29,118,26,18,59,273,34,19,14,041,,2*7D\r\n$GAGSV,3,3,09,36,38,315,18,2*4F\r\n$GBGSV,5,1,17,01,42,153,,03,45,207,,04,35,133,,05,09,257,,1*7C\r\n$GBGSV,5,2,17,06,29,183,,07,07,201,,08,66,358,34,09,09,195,,1*7F\r\n$GBGSV,5,3,17,10,14,222,23,11,34,144,21,13,51,316,,14,73,036,35,1*74\r\n$GBGSV,5,4,17,16,25,186,31,27,11,317,,28,62,307,38,33,76,249,30,1*70\r\n$GBGSV,5,5,17,34,10,143,,1*40\r\n$GBGSV,5,1,17,01,42,153,,03,45,207,,04,35,133,,05,09,257,,3*7E\r\n$GBGSV,5,2,17,06,29,183,,07,07,201,,08,66,358,41,09,09,195,,3*7F\r\n$GBGSV,5,3,17,10,14,222,,11,34,144,28,13,51,316,,14,73,036,43,3*7F\r\n$GBGSV,5,4,17,16,25,186,32,27,11,317,,28,62,307,,33,76,249,,3*79\r\n$GBGSV,5,5,17,34,10,143,,3*42\r\n$GNGLL,3723.59840,N,12656.92439,E,065307.00,A,A*76\r\n$GNRMC,065308.00,A,3723.59854,N,12656.92439,E,0.023,,250720,,,A,V*1C\r\n$GNVTG,,T,,M,0.023,N,0.042,K,A*3A\r\n$GNGGA,065308.00,3723.59854,N,12656.92439,E,1,12,0.78,40.9,M,18.5,M,,*74\r\n$GNGSA,A,3,29,17,19,06,12,05,02,09,,,,,1.20,0.78,0.92,1*08\r\n$GNGSA,A,3,85,71,72,,,,,,,,,,1.20,0.78,0.92,2*0B\r\n$GNGSA,A,3,36,19,11,04,09,12,,,,,,,1.20,0.78,0.92,3*07\r\n$GNGSA,A,3,28,11,14,10,33,08,,,,,,,1.20,0.78,0.92,4*05\r\n$GPGSV,4,1,13,02,69,341,34,04,05,036,07,05,51,267,38,06,55,084,35,1*69\r\n$GPGSV,4,2,13,07,08,101,,09,35,053,35,12,16,259,26,13,12,191,18,1*6F\r\n$GPGSV,4,3,13,17,14,158,16,19,32,163,36,25,10,289,22,29,11,322,23,1*6D\r\n$GPGSV,4,4,13,30,04,130,,1*53\r\n$GPGSV,4,1,13,02,69,341,,04,05,036,,05,51,267,33,06,55,084,37,6*67\r\n$GPGSV,4,2,13,07,08,101,,09,35,053,38,12,16,259,,13,12,191,,6*68\r\n$GPGSV,4,3,13,17,14,158,,19,32,163,,25,10,289,17,29,11,322,18,6*66\r\n$GPGSV,4,4,13,30,04,130,,6*54\r\n$GLGSV,2,1,06,70,49,030,,71,73,235,35,72,22,219,29,84,04,137,08,1*75\r\n$GLGSV,2,2,06,85,59,121,31,86,57,339,,1*7A\r\n$GLGSV,2,1,06,70,49,030,,71,73,235,39,72,22,219,21,84,04,137,12,3*78\r\n$GLGSV,2,2,06,85,59,121,31,86,57,339,,3*78\r\n$GAGSV,3,1,09,02,02,284,10,04,67,075,29,05,01,213,,09,48,198,35,7*7C\r\n$GAGSV,3,2,09,11,78,057,27,12,29,118,25,18,59,273,43,19,14,041,16,7*7F\r\n$GAGSV,3,3,09,36,38,315,27,7*46\r\n$GAGSV,3,1,09,02,02,284,,04,67,075,39,05,01,213,,09,48,198,33,2*7F\r\n$GAGSV,3,2,09,11,78,057,36,12,29,118,26,18,59,273,33,19,14,041,,2*79\r\n$GAGSV,3,3,09,36,38,315,19,2*4E\r\n"
  in  "clear":bool
  out "wgs84":cluster{dbl, dbl}={12656.92439, 3723.59854}
